vi "get Main Texture Name.vi"(11 "Element in":refnum<class "Element.lvclass">) -> (3 "Main Texture Name":string)   [LabVIEW 2021, in "Element.lvclass"]
uses:
  Element.lvclass
  Element.lvclass/Element.ctl
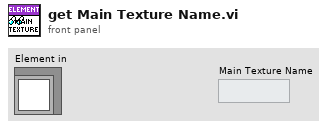
[diagram p1: front panel]
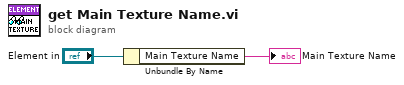
[diagram p0: block diagram]
diagram:
  n1 = Unbundle By Name("Element in") -> ("Main Texture Name"=→"Main Texture Name":string)
